vi "Actor Core.vi"(8 "Error In":errorcluster, 11 "CS++ObjectManager in":refnum<class "CS++ObjectManager.lvclass">) -> (0 "Error Out":errorcluster, 3 "Actor out":refnum<class "Actor.lvclass">)   [LabVIEW 2016, in "CS++ObjectManager.lvlib" / "CS++ObjectManager.lvclass"]
doc: "(<B>Filename</B>: Actor Framework.lvlib:Actor.lvclass:Actor Core.vi)\n\nReceives messages to the actor, reacts to them, and initiates any error handling that may shut the actor down.\n\nDescendant classes may override this VI to append parallel tasks for the actor to complete while it handles messages. Overrides use the Call Parent Method node."
uses:
  CS++ObjectManager.lvclass
  C:/User/Brand/LVP/TASCA/UTCS/Packages/CSPP_Core/Actors/CS++BaseActor/CS++BaseActor.lvclass
  C:/User/Brand/LVP/TASCA/UTCS/Packages/CSPP_Core/Actors/CS++GUIActor/CS++GUIActor.lvclass
  C:/Program Files (x86)/National Instruments/LabVIEW 2016/vi.lib/ActorFramework/Actor/Actor.lvclass
  <vilib>/ActorFramework/Actor/Actor.lvclass
  CSPP_Core/Actors/CS++BaseActor/CS++BaseActor.lvclass/CS++BaseActor.ctl
  <vilib>/ActorFramework/Message Enqueuer/Message Enqueuer.lvclass
  CS++ObjectManager.lvclass/CS++ObjectManager.ctl
  CSPP_Core/Actors/CS++GUIActor/CS++GUIActor.lvclass/CS++GUIActor.ctl
  <vilib>/ActorFramework/Actor/Actor.lvclass/Actor.ctl
  <vilib>/ActorFramework/Message Enqueuer/Message Enqueuer.lvclass/Message Enqueuer.ctl
  CSPP_Core/Libraries/Base/FGV Action.ctl
  CSPP_Core/Actors/CS++StartActor Messages/Launch Actors Msg/Launch Actors Msg.lvclass/Launch Actors Msg.ctl
  CS++ObjectManager Messages/Write Actor Filter Msg/Write Actor Filter Msg.lvclass/Write Actor Filter Msg.ctl
  <vilib>/ActorFramework/Message/Message.lvclass
  CSPP_Core/Actors/CS++BaseActor Messages/Launch Associated GUI Msg/Launch Associated GUI Msg.lvclass
  C:/Program Files (x86)/National Instruments/LabVIEW 2016/vi.lib/ActorFramework/Message/Message.lvclass
  CSPP_Core/Actors/CS++BaseActor Messages/Open Actor Core FP Msg/Open Actor Core FP Msg.lvclass/Open Actor Core FP Msg.ctl
  CSPP_Core/Actors/CS++BaseActor/Read Object Name.vi
  CSPP_Core/Actors/CS++GUIActor/Read Stop-Event.vi
  CSPP_Core/Actors/CS++GUIActor/Read PV-Update.vi
  <vilib>/ActorFramework/Message Enqueuer/Init from Existing Queue.vi
  <vilib>/ActorFramework/Stop Msg/Stop Msg.lvclass
  CSPP_Core/Actors/CS++StartActor Messages/Launch Actors Msg/Launch Actors Msg.lvclass
  CSPP_Core/Actors/CS++StartActor Messages/Read Actor List Msg/Read Actor List Msg.lvclass
  CS++ObjectManager Messages/Update Actor List Msg/Update Actor List Msg.lvclass
  CS++ObjectManager Messages/Write Actor Filter Msg/Write Actor Filter Msg.lvclass
  CSPP_Core/Actors/CS++BaseActor Messages/Open Actor Core FP Msg/Open Actor Core FP Msg.lvclass
  <vilib>/ActorFramework/Message Priority Queue/Priority Enqueue.vi
  CSPP_Core/Classes/CS++ProcessVariables/ProcessVariable/PV.lvclass
  CSPP_Core/Classes/CS++BaseClasses/Factory/CS++Factory.lvclass
  CSPP_Core/Actors/CS++GUIActor/CS++GUIActor.lvclass
  CSPP_Core/Actors/CS++BaseActor/CS++BaseActor.lvclass
  CSPP_Core/Libraries/Base/CS++Base.lvlib
panel:
  in  "Actor List":i32(listbox)
  in  "Stop Button":bool
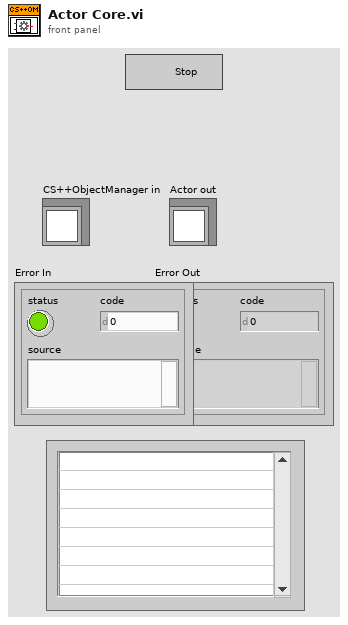
[diagram p1: front panel]
types:
  T1 = enum32{"Invalid", "Standard", "Closed", "Hidden", "Minimized", "Maximized"}
  T2 = typedef "CS++Base.lvlib/FGV Action.ctl" = enum16{"add", "replace", "read", "remove", "reset", "get attributes"}
  T3 = cluster{"Class Name":string, "Enqueuer":refnum<class "Message Enqueuer.lvclass">}[]
  T4 = typedef "LVMenuShortCut.ctl" = cluster{"include Shift key?":bool, "include Ctrl key?":bool, "shortcut key":string}
  T5 = cluster{"Class Name":string, "Enqueuer":refnum<class "Message Enqueuer.lvclass">}
  T6 = cluster{"PVMonitor":bool, "PVProxy":bool, "GUI":bool, "Other":bool}
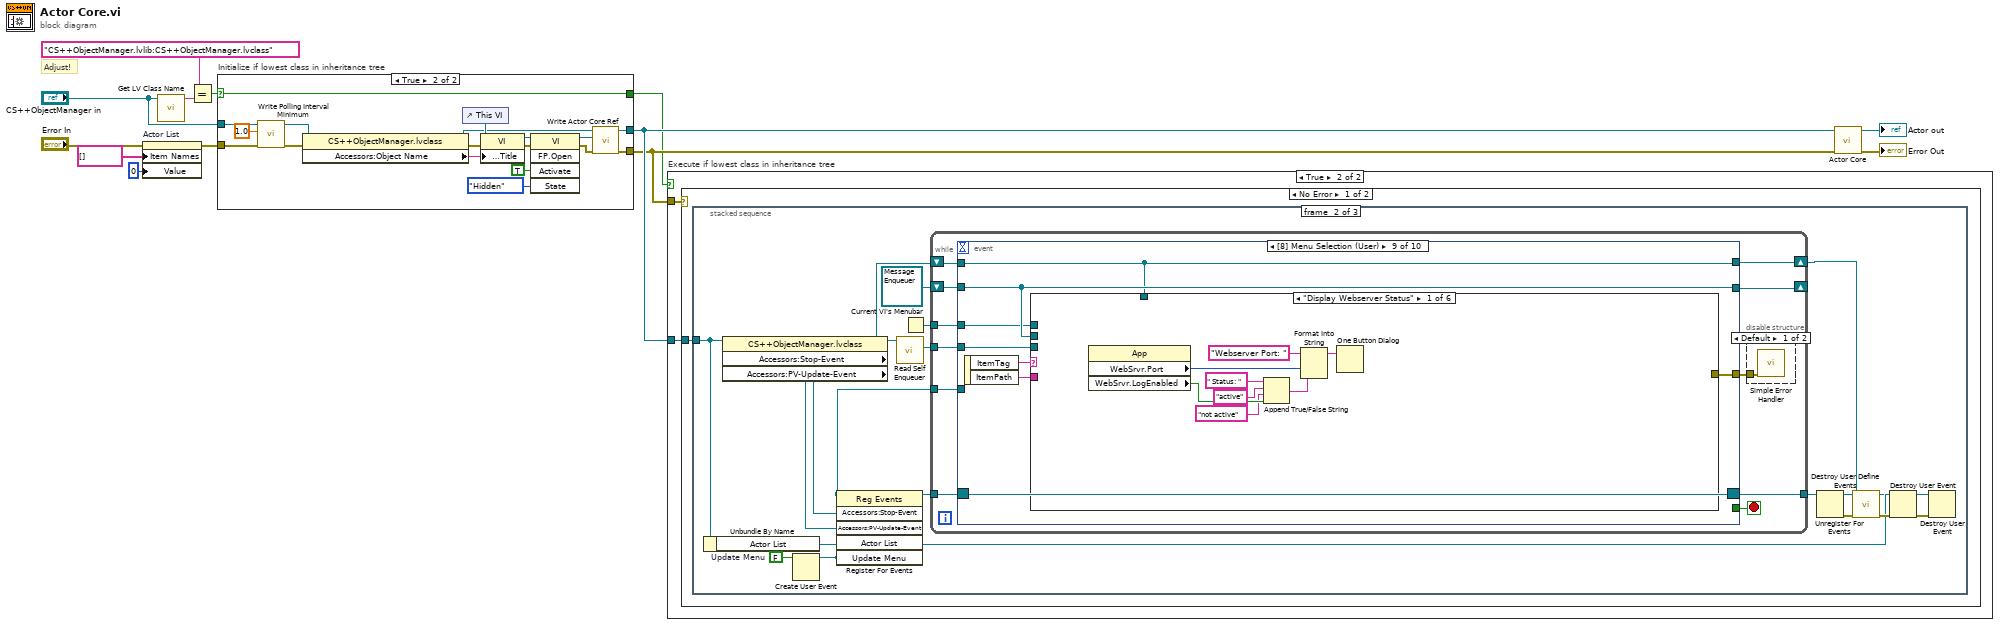
[diagram p0: block diagram]
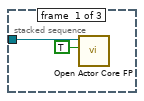
[diagram p3: hidden frame]
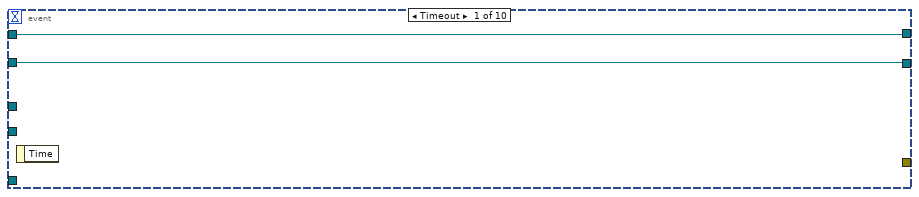
[diagram p5: hidden frame]
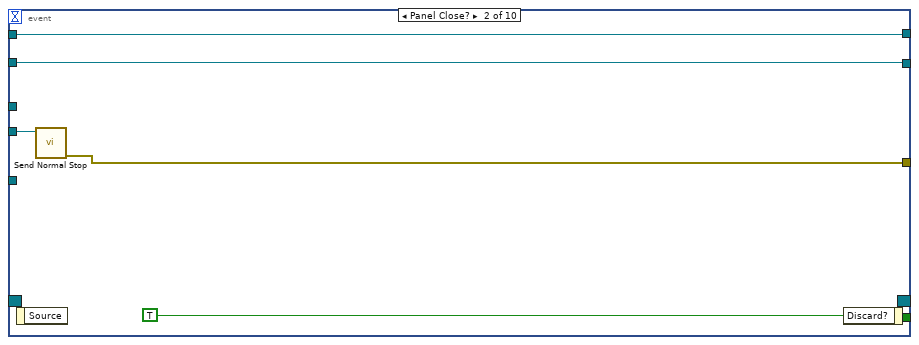
[diagram p6: hidden frame]
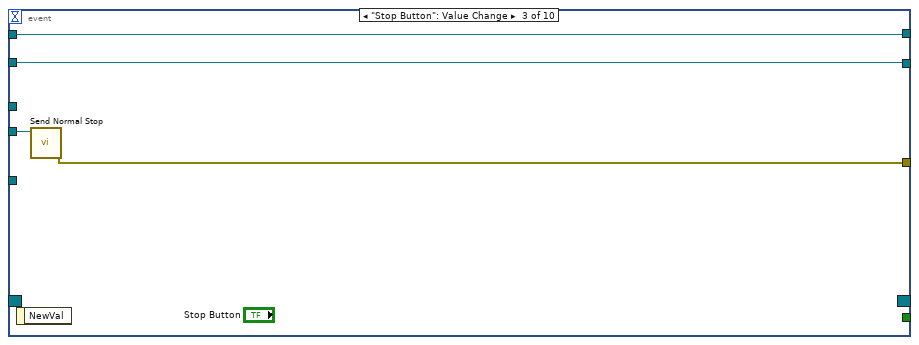
[diagram p7: hidden frame]
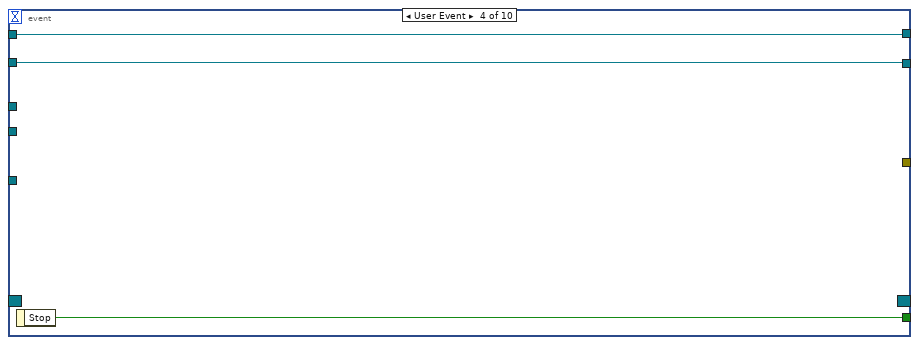
[diagram p8: hidden frame]
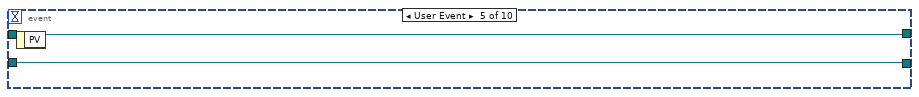
[diagram p9: hidden frame]
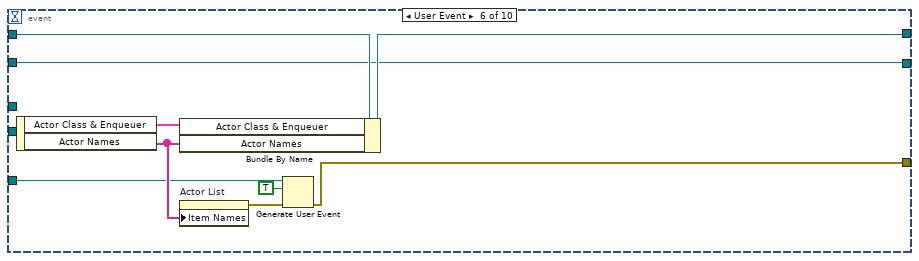
[diagram p10: hidden frame]
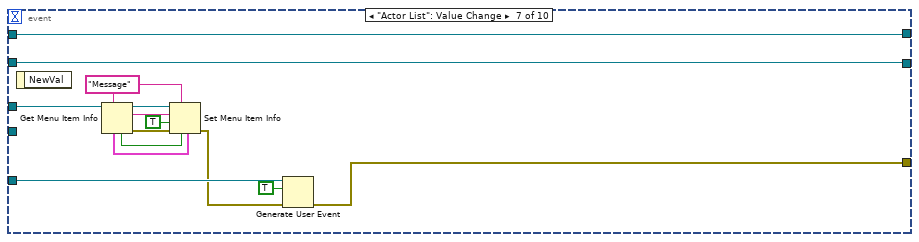
[diagram p11: hidden frame]
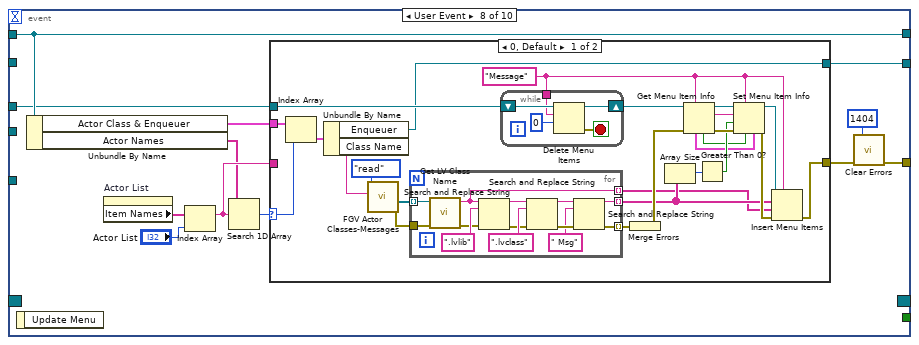
[diagram p12: hidden frame]
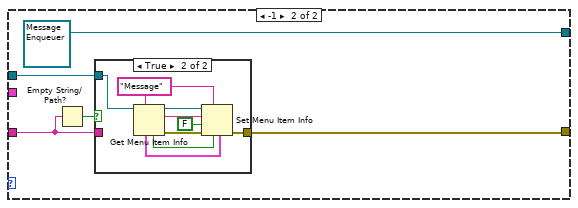
[diagram p13: hidden frame]
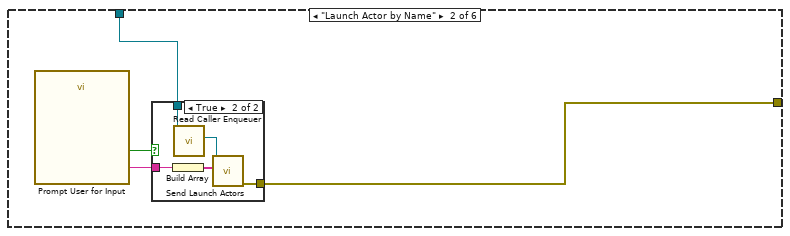
[diagram p15: hidden frame]
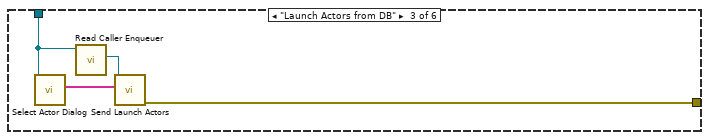
[diagram p17: hidden frame]
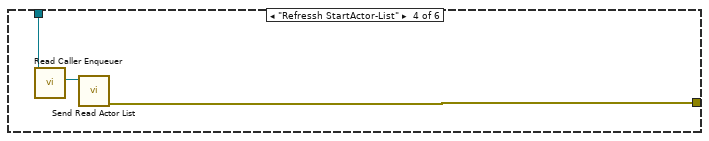
[diagram p18: hidden frame]
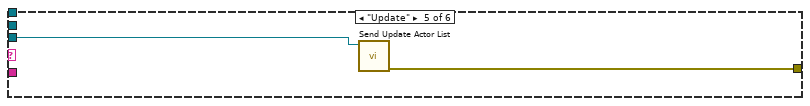
[diagram p19: hidden frame]
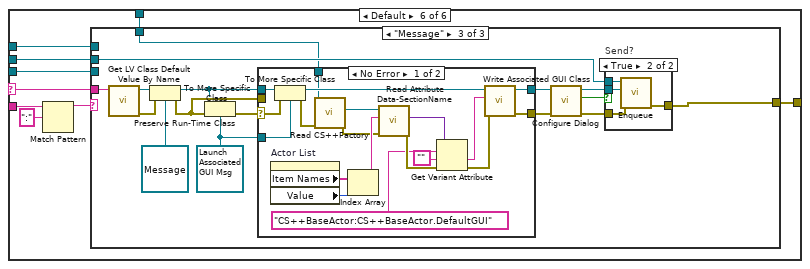
[diagram p20: hidden frame]
diagram:
  # "Adjust!"
  n1 = property on="Actor List" class="LstBox (strict)"(error in="Error In", "Item Names"=string[] [], "Value"=0 ("Actor List")) -> (error out=w2:errorcluster)  [unwired: 1 in, 1 out]
  n2 = call <vilib>:"Get LV Class Name.vi"("object"="CS++ObjectManager in") -> ("class name"=w13:string)  [unwired: 9 in, 1 out]
  n3 = Equal?(x="CS++ObjectManager.lvlib:CS++ObjectManager.lvclass" ("class name"), y=w13) -> (x = y?=w9:bool)
  n4 = case "Initialize if lowest class in inheritance tree" shown="True" w9 {
    selector: w9 -> [w16 w32]
    tunnel: w2 -> [w14 w19]
    tunnel: "CS++ObjectManager in" -> [w15 w21]
    tunnel: [w15 w29] -> w11
    tunnel: [w14 w28] -> w10
    tunnel: [w16 w32] -> w8
    frame False {
    }
    frame True {
      n5 = call "Write Polling Interval Minimum.vi"("error in (no error)"=w19, "Polling Interval Minimum"=dbl[unit] 1.0, "CS++BaseActor in"=w21) -> ("error out"=w18:errorcluster, "CS++BaseActor out"=w20:refnum<class "CS++ObjectManager.lvclass">)  [unwired: 7 in]
      n6 = property class="CS++ObjectManager.lvclass"(reference=w20, error in=w18) -> (reference out=w22:refnum<class "CS++ObjectManager.lvclass">, error out=w24:errorcluster, "Accessors:Object Name"=w23:string)
      n7 = control-ref of="This VI"() -> (w27:refnum<vi>)
      n8 = property class="VI"(reference=w27, error in=w24, "Front Panel.Title"=w23) -> (reference out=w26:refnum<vi>, error out=w25:errorcluster)
      n9 = invoke class="VI" method="FP.Open"(reference=w26, error in=w25, "Activate"=TRUE ("Activate?"), "State"=T1."Hidden") -> (reference out=w31:refnum<vi>, error out=w30:errorcluster)  [unwired: 1 in, 3 out]
      n10 = call "Write Actor Core Ref.vi"("error in (no error)"=w30, "Actor Core Ref"=w31, "CS++BaseActor in"=w22) -> ("error out"=w28:errorcluster, "CS++BaseActor out"=w29:refnum<class "CS++ObjectManager.lvclass">)  [unwired: 7 in]
    }
  }
  n11 = case "Execute if lowest class in inheritance tree" shown="True" w8 {
    tunnel: w11 -> [_ w36]
    tunnel: w10 -> [_ w35]
    frame False {
    }
    frame True {
      n12 = case shown="No Error" w35 {
        tunnel: w36 -> [w37 _]
        frame No Error {
          n13 = stacked-sequence {
            tunnel: w37 -> [w39 w47 w361]
            frame #0 {
              n14 = call "Open Actor Core FP.vi"("Open FP (F)"=TRUE, "CS++BaseActor in"=w39) -> ()  [unwired: 8 in, 2 out]
            }
            frame #1 {
              w44 = FALSE  # Update Menu
              n15 = Unbundle By Name(w47) -> ("Actor List"=w45:refnum<user-event>)
              n16 = property class="CS++ObjectManager.lvclass"(reference=w47) -> (reference out=w49:refnum<class "CS++ObjectManager.lvclass">, "Accessors:Stop-Event"=w51:refnum<user-event>, "Accessors:PV-Update-Event"=w50:refnum<user-event>)  [unwired: 1 in, 1 out]
              n17 = Create User Event(user event datatype=w44) -> (user event=w42:refnum<user-event>)  [unwired: 1 in, 1 out]
              n18 = register-events(w51, w50, w45, w42) -> (reference out=w52:refnum<event-registration>)  [unwired: 2 in, 1 out]
              n19 = call <vilib>:"Read Self Enqueuer.vi"("Actor"=w49) -> ("Self Enqueuer"=w53:refnum<class "Message Enqueuer.lvclass">)  [unwired: 10 in]
              n20 = Current VI's Menubar() -> (w41:refnum<k9>)
              n21 = while {
                tunnel: w52 -> [w66]
                tunnel: [w64] -> w55
                tunnel: w53 -> [w62]
                shift-right: [w60] -> w48
                shift-left: w49 -> [w61]
                tunnel: w42 -> [w59]
                tunnel: w41 -> [w58]
                shift-right: [w57] -> _
                shift-left: refnum<class "Message Enqueuer.lvclass"> refnum ("Enqueuer") -> [w56]
                stop <- w65 stop-if-true
                n22 = event shown="[8] Menu Selection (User)" {
                  selector: w66 -> [_ _ _ _ _ _ _ _ _ _]
                  dyn-events: [_ _ _ _ _ _ _ _ _ _] -> w64
                  timeout: _ -> [_ _ _ _ _ _ _ _ _ _]
                  tunnel: [_ _ _ w81 _ _ _ _ _ _] -> w65
                  tunnel: [_ w73 w78 _ _ w86 w103 w109 w181 w313] -> w63
                  tunnel: w62 -> [_ w72 w77 _ _ _ _ _ w182 _]
                  tunnel: [w69 w71 w76 w80 w83 w91 w106 w113 w176 w311] -> w60
                  tunnel: w61 -> [w69 w71 w76 w80 w83 w92 w106 w113 w176 w311]
                  tunnel: w59 -> [_ _ _ _ _ w87 w104 _ _ _]
                  tunnel: w58 -> [_ _ _ _ _ _ w101 w111 w177 _]
                  tunnel: [w68 w70 w75 w79 w82 w84 w102 w110 w178 w304] -> w57
                  tunnel: w56 -> [w68 w70 w75 w79 w82 w84 w102 _ w178 w304]
                  event Timeout {
                    n23 = event-data() -> ()  [unwired: 1 in, 1 out]
                  }
                  event Panel Close? {
                    n24 = event-data() -> ()  [unwired: 1 in, 1 out]
                    n25 = call <vilib>:"Send Normal Stop.vi"("Message Enqueuer"=w72) -> ("error out"=w73:errorcluster)  [unwired: 10 in]
                    n26 = event-data("Discard?"=TRUE) -> ()  [unwired: 1 in, 1 out]
                  }
                  event "Stop Button": Value Change {
                    n27 = event-data() -> ()  [unwired: 1 in, 1 out]
                    n28 = call <vilib>:"Send Normal Stop.vi"("Message Enqueuer"=w77) -> ("error out"=w78:errorcluster)  [unwired: 10 in]
                  }
                  event User Event {
                    n29 = event-data() -> ("Stop"=w81:bool)  [unwired: 1 in]
                  }
                  event User Event {
                    n30 = event-data() -> ()  [unwired: 1 in, 1 out]
                  }
                  event User Event {
                    n31 = event-data() -> ("Actor Class & Enqueuer"=w88:T3, "Actor Names"=w90:string[])  [unwired: 1 in]
                    n32 = Bundle By Name(cluster=w92, "Actor Class & Enqueuer"=w88, "Actor Names"=w90) -> (w91:refnum<class "CS++ObjectManager.lvclass">)
                    n33 = property on="Actor List" class="LstBox (strict)"("Item Names"=w90) -> (error out=w89:errorcluster)  [unwired: 2 in, 1 out]
                    n34 = Generate User Event(user event=w87, event data cluster=TRUE ("event data"), error in=w89) -> (error out=w86:errorcluster)  [unwired: 1 in, 1 out]
                  }
                  event "Actor List": Value Change {
                    w98 = "Message" ("item tag")
                    n35 = event-data() -> ()  [unwired: 1 in, 1 out]
                    n36 = Get Menu Item Info(7:w98, 11:w101) -> (0:w99:errorcluster, 2:w97:string, 3:w100:refnum<k9>, 4:w96:bool, 6:w95:T4)  [unwired: 1 in, 2 out]
                    n37 = Set Menu Item Info(4:w95, 6:w96, 7:w98, 8:w99, 9:TRUE ("enabled"), 10:w97, 11:w100) -> (0:w93:errorcluster)  [unwired: 1 out]
                    n38 = Generate User Event(user event=w104, event data cluster=TRUE ("event data"), error in=w93) -> (error out=w103:errorcluster)  [unwired: 1 in, 1 out]
                  }
                  event User Event {
                    n39 = event-data() -> ()  [unwired: 1 in, 1 out]
                    n40 = Unbundle By Name(w113) -> ("Actor Class & Enqueuer"=w115:T3, "Actor Names"=w116:string[])
                    n41 = property on="Actor List" class="LstBox (strict)"() -> ("Item Names"=w114:string[])  [unwired: 2 in, 2 out]
                    n42 = Index Array(array=w114, index="Actor List") -> (element=w118:string)
                    n43 = Search 1D Array(1D array=w116, element=w118) -> (index of element=w117:i32)  [unwired: 1 in]
                    n44 = case shown="0, Default" w117 {
                      selector: w117 -> [w142 _]
                      tunnel: w115 -> [w143 _]
                      tunnel: w118 -> [_ w165]
                      tunnel: w111 -> [w127 w163]
                      tunnel: [w124 w162] -> w108
                      tunnel: [w119 refnum<class "Message Enqueuer.lvclass"> refnum ("Enqueuer")] -> w110
                      frame 0, Default {
                        w125 = "Message" ("menu tag")
                        n45 = Index Array(array=w143, index=w142) -> (element=w141:T5)
                        n46 = Unbundle By Name(w141) -> ("Enqueuer"=w119:refnum<class "Message Enqueuer.lvclass">, "Class Name"=w140:string)
                        n47 = call "FGV Actor Classes-Messages.vi"("Class Name"=w140, "Action (read)"=FGV_Action."read") -> ("Error Out"=w137:errorcluster, "CS++Messages"=w138:refnum<class "Message.lvclass">[])  [unwired: 5 in, 3 out]
                        n48 = for {
                          tunnel: w138 -> [w161] mode=indexing
                          tunnel: w137 -> [w160]
                          tunnel: [w153] -> w121 mode=indexing
                          tunnel: [w149] -> w123 mode=indexing
                          tunnel: [w154] -> w120 mode=indexing
                          n49 = call <vilib>:"Get LV Class Name.vi"("error in (no error)"=w160, "object"=w161) -> ("error out"=w156:errorcluster, "class name"=w154:string)  [unwired: 8 in]
                          n50 = Search and Replace String(input string=w154, search string=".lvlib", error in=w156) -> (result string=w157:string, error out=w155:errorcluster)  [unwired: 5 in, 2 out]
                          n51 = Search and Replace String(input string=w157, search string=".lvclass", error in=w155) -> (result string=w152:string, error out=w151:errorcluster)  [unwired: 5 in, 2 out]
                          n52 = Search and Replace String(input string=w152, search string=" Msg", error in=w151) -> (result string=w153:string, error out=w149:errorcluster)  [unwired: 5 in, 2 out]
                        }
                        n53 = while {
                          tunnel: w125 -> [w146]
                          shift-right: [w147] -> w126
                          shift-left: w127 -> [w148]
                          stop <- w144 stop-if-true
                          n54 = Delete Menu Items(7:0, 8:w146, 9:w148) -> (0:w144:errorcluster, 3:w147:refnum<k9>)  [unwired: 1 in]
                        }
                        n55 = Merge Errors(w123) -> (w122:errorcluster)
                        n56 = Array Size(array=w121) -> (size(s)=w133:i32)
                        n57 = Get Menu Item Info(7:w125, 8:w122, 11:w126) -> (0:w136:errorcluster, 2:w134:string, 3:w135:refnum<k9>, 4:w131:bool, 6:w130:T4)  [unwired: 2 out]
                        n58 = Greater Than 0?(x=w133) -> (x > 0?=w132:bool)
                        n59 = Set Menu Item Info(4:w130, 6:w131, 7:w125, 8:w136, 9:w132, 10:w134, 11:w135) -> (0:w128:errorcluster, 3:w129:refnum<k9>)
                        n60 = Insert Menu Items(5:w125, 6:w128, 7:w120, 8:w121, 9:w129) -> (0:w124:errorcluster)  [unwired: 1 in, 2 out]
                      }
                      frame -1 {
                        n61 = Empty String/Path?(string/path=w165) -> (empty?=w164:bool)
                        n62 = case shown="True" w164 {
                          tunnel: w165 -> [_ _]
                          tunnel: w163 -> [_ w168]
                          tunnel: [_ w167] -> w162
                          frame False {
                          }
                          frame True {
                            w173 = "Message" ("item tag")
                            n63 = Get Menu Item Info(7:w173, 11:w168) -> (0:w174:errorcluster, 2:w172:string, 3:w175:refnum<k9>, 4:w171:bool, 6:w170:T4)  [unwired: 1 in, 2 out]
                            n64 = Set Menu Item Info(4:w170, 6:w171, 7:w173, 8:w174, 9:FALSE ("enabled"), 10:w172, 11:w175) -> (0:w167:errorcluster)  [unwired: 1 out]
                          }
                        }
                      }
                    }
                    n65 = call <vilib>:"Clear Errors.vi"("error in (no error)"=w108, "specific error code to clear (0: all)"=1404) -> ("error out"=w109:errorcluster)  [unwired: 4 in, 1 out]
                  }
                  event Menu Selection (User) {
                    n66 = event-data() -> ("ItemTag"=w180:string, "ItemPath"=w179:string)  [unwired: 1 in]
                    n67 = case shown="\"Display Webserver Status\"" w180 {
                      selector: w180 -> [_ _ _ _ _ w214]
                      tunnel: w182 -> [_ _ _ _ w208 w211]
                      tunnel: [_ w193 w200 w204 w207 w212] -> w181
                      tunnel: w179 -> [_ _ _ _ _ w217]
                      tunnel: w178 -> [_ _ _ _ _ w213]
                      tunnel: w177 -> [_ _ _ _ _ w210]
                      tunnel: w176 -> [_ w194 w202 w206 _ w209]
                      frame "Display Webserver Status" {
                        n68 = property class="App"() -> ("WebSrvr.Port"=w190:u16, "WebSrvr.LogEnabled"=w188:bool)  [unwired: 2 in, 2 out]
                        n69 = Append True/False String(1:w188, 2:"not active" ("true string"), 3:"active" ("true string"), 4:" Status: " ("string (\"\")")) -> (0:w186:string)
                        n70 = Format Into String(initial string="Webserver Port: ", w190, w186) -> (resulting string=w183:string)  [unwired: 2 in, 1 out]
                        n71 = One Button Dialog(message=w183) -> ()  [unwired: 1 in, 1 out]
                      }
                      frame "Launch Actor by Name" {
                        n72 = call "Prompt User for Input"() -> ("Name"=w192:string, "Launch"=w191:bool)  [unwired: 17 in, 1 out]
                        n73 = case shown="True" w191 {
                          tunnel: w194 -> [_ w199]
                          tunnel: [_ w197] -> w193
                          tunnel: w192 -> [_ w196]
                          frame False {
                          }
                          frame True {
                            n74 = Build Array(w196) -> (w195:string[])
                            n75 = call <vilib>:"Read Caller Enqueuer.vi"("Actor"=w199) -> ("Caller Enqueuer"=w198:refnum<class "Message Enqueuer.lvclass">)  [unwired: 10 in]
                            n76 = call "Send Launch Actors.vi"("Selected Actors"=w195, "Message Enqueuer"=w198) -> ("error out"=w197:errorcluster)  [unwired: 8 in, 1 out]
                          }
                        }
                      }
                      frame "Launch Actors from DB" {
                        n77 = call "Select Actor Dialog.vi"("CS++ObjectManager"=w202) -> ("Selected Names"=w203:string[])  [unwired: 8 in, 2 out]
                        n78 = call <vilib>:"Read Caller Enqueuer.vi"("Actor"=w202) -> ("Caller Enqueuer"=w201:refnum<class "Message Enqueuer.lvclass">)  [unwired: 10 in]
                        n79 = call "Send Launch Actors.vi"("Selected Actors"=w203, "Message Enqueuer"=w201) -> ("error out"=w200:errorcluster)  [unwired: 8 in, 1 out]
                      }
                      frame "Refressh StartActor-List" {
                        n80 = call <vilib>:"Read Caller Enqueuer.vi"("Actor"=w206) -> ("Caller Enqueuer"=w205:refnum<class "Message Enqueuer.lvclass">)  [unwired: 10 in]
                        n81 = call "Send Read Actor List.vi"("Message Enqueuer"=w205) -> ("error out"=w204:errorcluster)  [unwired: 9 in, 1 out]
                      }
                      frame "Update" {
                        n82 = call "Send Update Actor List.vi"("Message Enqueuer"=w208) -> ("error out"=w207:errorcluster)  [unwired: 9 in, 1 out]
                      }
                      frame Default {
                        n83 = Match Pattern(string=w217, regular expression=":") -> (before substring=w215:string)  [unwired: 1 in, 3 out]
                        n84 = case shown="\"Message\"" w215 {
                          selector: w215 -> [_ w241 _]
                          tunnel: w214 -> [_ w224 w277]
                          tunnel: w213 -> [_ _ w273]
                          tunnel: [_ w229 w272] -> w212
                          tunnel: w211 -> [_ w233 _]
                          tunnel: w210 -> [_ w220 _]
                          tunnel: w209 -> [_ w236 w264]
                          frame Default {
                          }
                          frame "View" {
                            n85 = Get Menu Item Info(7:w224, 11:w220) -> (0:w227:errorcluster, 1:w225:bool, 2:w226:string, 3:w228:refnum<k9>, 4:w222:bool, 6:w223:T4)  [unwired: 1 in, 1 out]
                            n86 = Unbundle By Name(w236) -> ("Actor Filter"=w235:T6)
                            n87 = Not(x=w222) -> (.not. x?=w221:bool)
                            n88 = Set Menu Item Info(4:w223, 6:w221, 7:w224, 8:w227, 9:w225, 10:w226, 11:w228) -> (0:w218:errorcluster, 3:w219:refnum<k9>)
                            n89 = Get Menu Item Info(7:w241, 8:w218, 11:w219) -> (0:w238:errorcluster, 3:w239:refnum<k9>, 5:w240:string[])  [unwired: 4 out]
                            n90 = for {
                              tunnel: w240 -> [w242] mode=indexing
                              tunnel: w239 -> [w248]
                              tunnel: w238 -> [w247]
                              tunnel: [w246] -> w237 mode=indexing
                              shift-right: [w243] -> w234
                              shift-left: w235 -> [w245]
                              n91 = Get Menu Item Info(7:w242, 8:w247, 11:w248) -> (0:w246:errorcluster, 4:w244:bool)  [unwired: 5 out]
                              n92 = case shown="\"Other\"" w242 {
                                tunnel: w245 -> [w249 w252 w255 w258 w261]
                                tunnel: w244 -> [_ w251 w254 w257 w260]
                                tunnel: [w249 w250 w253 w256 w259] -> w243
                                frame Default {
                                }
                                frame "PVMonitor" {
                                n93 = Bundle By Name(cluster=w252, "PVMonitor"=w251) -> (w250:T6)
                                }
                                frame "PVProxy" {
                                n94 = Bundle By Name(cluster=w255, "PVProxy"=w254) -> (w253:T6)
                                }
                                frame "GUI" {
                                n95 = Bundle By Name(cluster=w258, "GUI"=w257) -> (w256:T6)
                                }
                                frame "Other" {
                                n96 = Bundle By Name(cluster=w261, "Other"=w260) -> (w259:T6)
                                }
                              }
                            }
                            n97 = Merge Errors(w237) -> (w232:errorcluster)
                            n98 = call "Send Write Actor Filter.vi"("error in (no error)"=w232, "Actor Filter"=w234, "Message Enqueuer"=w233) -> ("error out"=w231:errorcluster, "Message Enqueuer out"=w230:refnum<class "Message Enqueuer.lvclass">)  [unwired: 7 in]
                            n99 = call "Send Update Actor List.vi"("error in (no error)"=w231, "Message Enqueuer"=w230) -> ("error out"=w229:errorcluster)  [unwired: 8 in, 1 out]
                          }
                          frame "Message" {
                            w266 = refnum<class "Launch Associated GUI Msg.lvclass"> refnum ("CS++BaseActor.lvlib:Launch Associated GUI Msg.lvclass")
                            n100 = call <vilib>:"Get LV Class Default Value By Name.vi"("class name"=w277) -> ("error out"=w275:errorcluster, "object"=w276:refnum<class>)  [unwired: 9 in]
                            n101 = To More Specific Class(target class=refnum<class "Message.lvclass"> refnum ("Actor Framework:Message"), reference=w276, error in=w275) -> (specific class reference=w262:refnum<class "Message.lvclass">, error out=w263:errorcluster)
                            n102 = Preserve Run-Time Class(object in=w262, error in=w263, 2:w266) -> (error out=w268:errorcluster)  [unwired: 1 out]
                            n103 = case shown="No Error" w268 {
                              selector: w268 -> [w294 _]
                              tunnel: [w292 w298] -> w267
                              tunnel: w262 -> [w296 w298]
                              tunnel: w266 -> [w295 _]
                              tunnel: [w291 w297] -> w265
                              tunnel: w264 -> [w287 _]
                              tunnel: w263 -> [_ w297]
                              frame No Error {
                                n104 = property on="Actor List" class="LstBox (strict)"() -> ("Item Names"=w290:string[], "Value"=w289:i32)  [unwired: 2 in, 2 out]
                                n105 = To More Specific Class(target class=w295, reference=w296, error in=w294) -> (specific class reference=w293:refnum<class "Launch Associated GUI Msg.lvclass">, error out=w286:errorcluster)
                                n106 = call "Read CS++Factory.vi"("error in (no error)"=w286, "CS++BaseActor in"=w287) -> ("error out"=w284:errorcluster, "CS++Factory"=w285:refnum<class "CS++Factory.lvclass">)  [unwired: 7 in, 1 out]
                                n107 = Index Array(array=w290, index=w289) -> (element=w288:string)
                                n108 = call-dynamic "Read Attribute Data-SectionName.vi"("error in (no error)"=w284, "Object Name"=w288, "CS++Factory in"=w285) -> ("error out"=w282:errorcluster, "Attribute Data"=w283:variant)  [unwired: 6 in, 1 out]
                                n109 = Get Variant Attribute(Variant=w283, name="CS++BaseActor:CS++BaseActor.DefaultGUI", default value (empty Variant)="", error in=w282) -> (value=w278:string, error out=w279:errorcluster)  [unwired: 2 out]
                                n110 = call-dynamic "Write Associated GUI Class.vi"("error in (no error)"=w279, "GUI Class"=w278, "Launch Associated GUI Msg in"=w293) -> ("error out"=w291:errorcluster, "Launch Associated GUI Msg out"=w292:refnum<class "Launch Associated GUI Msg.lvclass">)  [unwired: 7 in]
                              }
                              frame Error {
                              }
                            }
                            n111 = call-dynamic "Configure Dialog.vi"("Error In"=w265, "Message in"=w267) -> ("Error Out"=w271:errorcluster, "Ok?"=w269:bool, "Message out"=w270:refnum<class "Message.lvclass">)  [unwired: 7 in]
                            n112 = case "Send?" shown="True" w269 {
                              tunnel: w273 -> [_ w303]
                              tunnel: [w299 w302] -> w272
                              tunnel: w271 -> [w299 w301]
                              tunnel: w270 -> [_ w300]
                              frame False {
                              }
                              frame True {
                                n113 = call <vilib>:"Enqueue.vi"("error in (no error)"=w301, "Message"=w300, "Message Enqueuer in"=w303) -> ("error out"=w302:errorcluster)  [unwired: 7 in, 1 out]
                              }
                            }
                          }
                        }
                      }
                    }
                  }
                  event "Actor List": Shortcut Menu Selection (User) {
                    n114 = event-data() -> ("ItemTag"=w314:string, "CtlRef"=w312:refnum<vi>)  [unwired: 1 in]
                    n115 = Unbundle By Name(w311) -> ("Actor Class & Enqueuer"=w308:T3, "Actor Names"=w307:string[])
                    n116 = property class="LstBox (strict)"(reference=w312) -> ("Item Names"=w310:string[], "Value"=w309:i32)  [unwired: 1 in, 2 out]
                    n117 = Index Array(array=w310, index=w309) -> (element=w305:string)
                    n118 = Search 1D Array(1D array=w307, element=w305) -> (index of element=w306:i32)  [unwired: 1 in]
                    n119 = case shown="0, Default" w306 {
                      selector: w306 -> [w319 _]
                      tunnel: w314 -> [w322 _]
                      tunnel: [w321 _] -> w313
                      tunnel: w308 -> [w320 _]
                      tunnel: w305 -> [w315 w358]
                      frame 0, Default {
                        n120 = Index Array(array=w320, index=w319) -> (element=w318:T5)
                        n121 = Unbundle By Name(w318) -> ("Class Name"=w316:string, "Enqueuer"=w317:refnum<class "Message Enqueuer.lvclass">)
                        n122 = case shown="\"Stop\"" w322 {
                          tunnel: [_ w325 _ _ w347 w354] -> w321
                          tunnel: w317 -> [_ w323 _ _ w346 w353]
                          tunnel: w316 -> [_ _ w327 w336 _ _]
                          tunnel: w315 -> [_ _ w330 _ w344 w351]
                          frame Default {
                          }
                          frame "Open FP" {
                            n123 = call "Send Open Actor Core FP.vi"("Open FP (F)"=TRUE, "Message Enqueuer"=w323) -> ("error out"=w325:errorcluster)  [unwired: 8 in, 1 out]
                          }
                          frame "Display Class Name" {
                            w328 = "\r\n"
                            n124 = Concatenate Strings(w330, w328, "is instance of class" ("string"), w328, w327) -> (w326:string)
                            n125 = One Button Dialog(message=w326) -> ()  [unwired: 1 in, 1 out]
                          }
                          frame "Display Messages" {
                            n126 = call "FGV Actor Classes-Messages.vi"("Class Name"=w336, "Action (read)"=FGV_Action."read") -> ("Error Out"=w333:errorcluster, "CS++Messages"=w334:refnum<class "Message.lvclass">[])  [unwired: 5 in, 3 out]
                            n127 = for {
                              tunnel: w334 -> [w342] mode=indexing
                              tunnel: w333 -> [w341]
                              shift-right: [w338] -> w331
                              shift-left: "" -> [w340]
                              n128 = call <vilib>:"Get LV Class Name.vi"("error in (no error)"=w341, "object"=w342) -> ("class name"=w339:string)  [unwired: 8 in, 1 out]
                              n129 = Concatenate Strings(w340, "\r\n", w339) -> (w338:string)
                            }
                            n130 = One Button Dialog(message=w331) -> ()  [unwired: 1 in, 1 out]
                          }
                          frame "Stop" {
                            n131 = Two Button Dialog(message=w344, 2:"Stop Actor?" ("T button name (\"OK\")")) -> (T button?=w345:bool)  [unwired: 1 in]
                            n132 = case shown="True" w345 {
                              tunnel: [_ w349] -> w347
                              tunnel: w346 -> [_ w348]
                              frame False {
                              }
                              frame True {
                                n133 = call <vilib>:"Send Normal Stop.vi"("Message Enqueuer"=w348) -> ("error out"=w349:errorcluster)  [unwired: 10 in]
                              }
                            }
                          }
                          frame "Emergency Stop" {
                            n134 = Two Button Dialog(message=w351, 2:"Emergency Stop Actor?" ("T button name (\"OK\")")) -> (T button?=w352:bool)  [unwired: 1 in]
                            n135 = case shown="True" w352 {
                              tunnel: [_ w356] -> w354
                              tunnel: w353 -> [_ w355]
                              frame False {
                              }
                              frame True {
                                n136 = call <vilib>:"Send Normal Stop.vi"("Message Enqueuer"=w355) -> ("error out"=w356:errorcluster)  [unwired: 10 in]
                              }
                            }
                          }
                        }
                      }
                      frame -1 {
                        n137 = Concatenate Strings(w358, " not found in ist." ("string")) -> (w359:string)
                        n138 = One Button Dialog(message=w359) -> ()  [unwired: 1 in, 1 out]
                      }
                    }
                  }
                }
                n139 = disable-structure shown="Default" {
                  disable-tunnel: w63 -> [w67 _]
                  frame condition #0 (active) {
                    n140 = call <vilib>:"Simple Error Handler.vi"("error in (no error)"=w67) -> ()  [unwired: 4 in, 5 out]
                  }
                  frame condition #1 {
                  }
                }
              }
              n141 = Unregister For Events(event registration refnum=w55) -> (error out=w54:errorcluster)  [unwired: 1 in]
              n142 = call-dynamic "Destroy User Define Events.vi"("error in (no error)"=w54, "CS++GUIActor in"=w48) -> ("error out"=w46:errorcluster)  [unwired: 8 in, 1 out]
              n143 = Destroy User Event(user event=w45, error in=w46) -> (error out=w43:errorcluster)
              n144 = Destroy User Event(user event=w42, error in=w43) -> ()  [unwired: 1 out]
            }
            frame #2 {
              n145 = call "Open Actor Core FP.vi"("Open FP (F)"=FALSE, "CS++BaseActor in"=w361) -> ()  [unwired: 8 in, 2 out]
            }
          }
        }
        frame Error {
        }
      }
    }
  }
  n146 = call-parent "Actor Core.vi"("error in"=w10, "CS++GUIActor in"=w11) -> ("error out"=→"Error Out":errorcluster, "Actor out"=→"Actor out":refnum<class "Actor.lvclass">)  [unwired: 8 in]
